vi "add glyph core.vi"(6 "image data":T1, 8 "error in":errorcluster, 9 "name":string, 10 "base glyphs":T1[](array[typedef]), 11 "map in":variant) -> (0 "error out":errorcluster, 2 "base glyphs out":T1[](array[typedef]), 3 "map out":variant)   [LabVIEW 2025, in "CEF.lvlib"]
doc: "Copyright 2017 National Instruments Corporation\n\nLicensed under the Apache License, Version 2.0 (the \"License\"); you may not use this file except in compliance with the License. You may obtain a copy of the License at http://www.apache.org/licenses/LICENSE-2.0\nUnless required by applicable law or agreed to in writing, software distributed under the License is distributed on an \"AS IS\" BASIS, WITHOUT WARRANTIES OR CONDITIONS OF ANY KIND, either express or implied. See the License for the specific language governing permissions and limitations under the License."
uses:
  CEF.lvlib
  <vilib>/picture/picture.llb/imagedata.ctl
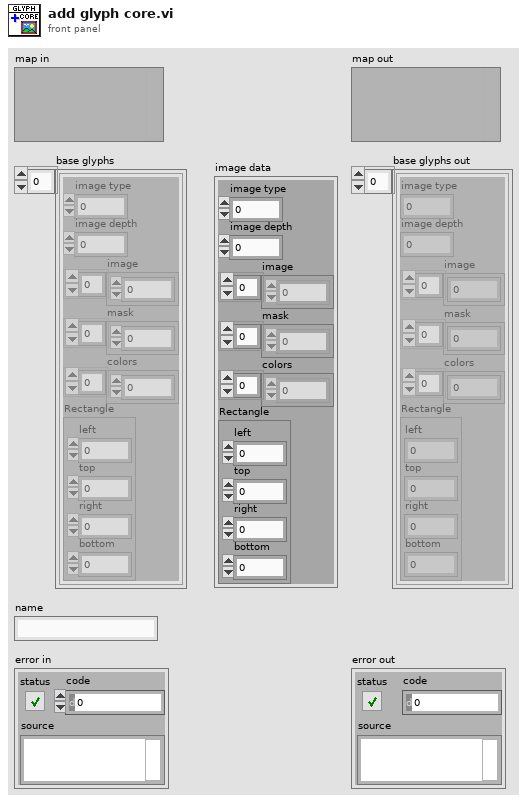
[diagram p1: front panel]
types:
  T1 = typedef "imagedata.ctl" = cluster{"image type":i32, "image depth":i32, "image":u8[], "mask":u8[], "colors":u32[], "Rectangle":cluster{"left":i16, "top":i16, "right":i16, "bottom":i16}}
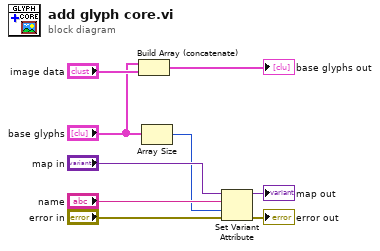
[diagram p0: block diagram]
diagram:
  n1 = Build Array (concatenate)("base glyphs", "image data") -> (→"base glyphs out":T1[])
  n2 = Array Size(array="base glyphs") -> (size(s)=w4:i32)
  n3 = Set Variant Attribute(Variant="map in", name="name", value=w4, error in="error in") -> (Variant out=→"map out":variant, error out=→"error out":errorcluster)  [unwired: 1 out]
